vi "LakeShore 370 Select Sensor.vi"(2 "Point #":i32, 3 "Parameters":dbl[](array[numeric]) format="%.3e", 4 "Instrument Address":refnum<visa-resource-name>) -> (0 "Stop":bool, 1 "Array":dbl[](array[numeric]) format="%.2f")   [LabVIEW 2020]
doc: "This VI changes the current channel on the LakeShore 370 Temperature contoller. The parameter is the channel to read. The stop always returns false.\nScott Hannahs, <sth@magnet.fsu.edu> NHMFL-FSU, May 2003"
panel:
  # "First parameter is the sensor number\nSecond parameter is the wait in seconds"
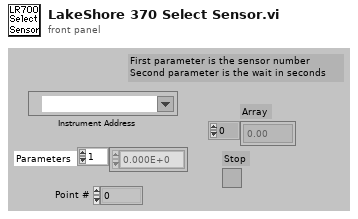
[diagram p1: front panel]
types:
  T1 = cluster{"Instrument":string, "ID Test String":string, "Terminator Character":string, u32, bool}
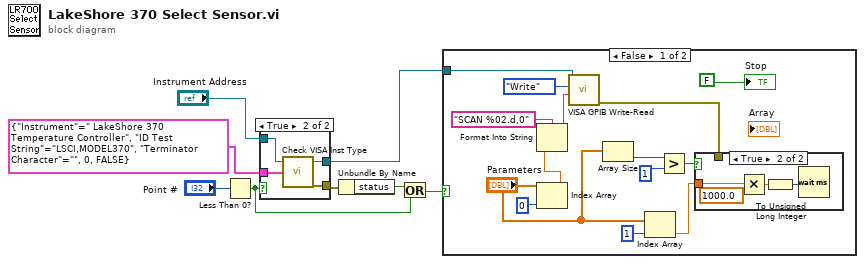
[diagram p0: block diagram]
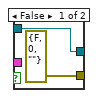
[diagram p4: hidden frame]
diagram:
  n1 = Less Than 0?(x="Point #") -> (x < 0?=w3:bool)
  n2 = case shown="True" w3 {
    tunnel: [w10 w13] -> w5
    tunnel: "Instrument Address" -> [w10 w12]
    tunnel: [errorcluster {"status"=FALSE, "code"=0, "source"=""} ("error out") w14] -> w8
    tunnel: T1 {"Instrument"=" LakeShore 370 Temperature Controller", "ID Test String"="LSCI,MODEL370", "Terminator Character"="", 0, FALSE} ("Instrument Info") -> [_ w11]
    frame False {
    }
    frame True {
      n3 = call "Check VISA Inst Type.vi"("Check Parameters"=w11, "VISA session"=w12) -> ("Error Out"=w14:errorcluster, "dup VISA session"=w13:refnum<visa-resource-name>)  [unwired: 1 in, 1 out]
    }
  }
  n4 = Unbundle By Name(w8) -> ("status"=w4:bool)
  n5 = Or(x=w4, y=w3) -> (x .or. y?=w2:bool)
  n6 = case shown="False" w2 {
    tunnel: w5 -> [w15 _]
    frame False {
      n7 = Index Array(array="Parameters", index=0) -> (element=w26:dbl)
      n8 = Format Into String(format string="SCAN %02.d,0", w26) -> (resulting string=w23:string)  [unwired: 2 in, 1 out]
      n9 = call "VISA GPIB Write-Read.vi"("Command"=w23, "Action"=enum16{"Write", "Read", "Write & Read"}."Write", "VISA resource name"=w15) -> ("error out"=w22:errorcluster)  [unwired: 5 in, 3 out]
      n10 = Array Size(array="Parameters") -> (size(s)=w20:i32)
      n11 = Index Array(array="Parameters", index=1) -> (element=w25:dbl)
      n12 = Greater?(x=w20, y=1) -> (0:w18:bool)
      n13 = case shown="True" w18 {
        tunnel: w25 -> [_ w31]
        tunnel: w22 -> [_ _]
        frame False {
        }
        frame True {
          n14 = Multiply(x=w31, y=1000.0) -> (x*y=w30:dbl)
          n15 = To Unsigned Long Integer(number=w30) -> (unsigned 32bit integer=w29:u32)
          n16 = Wait (ms)(milliseconds to wait=w29) -> ()  [unwired: 1 out]
        }
      }
      "Stop" <- FALSE
    }
    frame True {
    }
  }
